vi "Force Control Parameters DAO.vi"(7 "Config Ref Number":T2, 8 "error in (no error)":errorcluster, 9 "Force Control Parameters In":T1, 11 "DAO Actions":T3) -> (0 "error out":errorcluster, 2 "Force Control Parameters Out":T1, 4 "Config Ref Number out":T2)   [LabVIEW 2013]
uses:
  Metadata/Persistant DAO Actions.ctl
  <vilib>/Utility/config.llb/Config Data RefNum.ctl
  Force Control Parameters.ctl
  <vilib>/Utility/config.llb/Write Key (Boolean).vi
  <vilib>/Utility/config.llb/Write Key (I32).vi
  <vilib>/Utility/config.llb/Read Key (Boolean).vi
  <vilib>/Utility/config.llb/Read Key (I32).vi
  <vilib>/Utility/config.llb/NI_LVConfig.lvlib
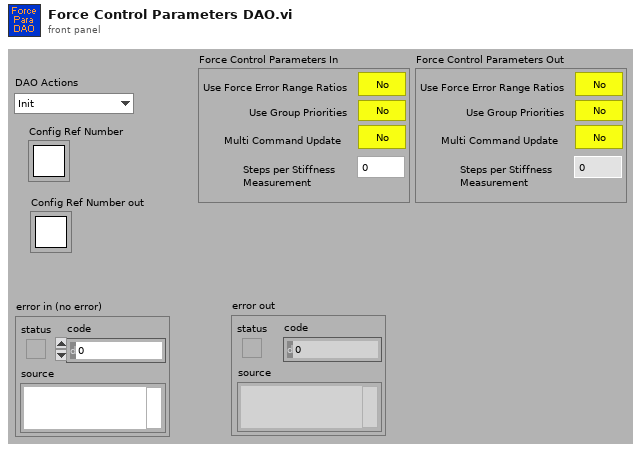
[diagram p1: front panel]
types:
  T1 = typedef "Force Control Parameters.ctl" = cluster{"Use Force Error Range Ratios":bool, "Use Group Priorities":bool, "Multi Command Update":bool, "Steps per Stiffness \nMeasurement":i32}
  T2 = typedef "NI_LVConfig.lvlib/Config Data RefNum.ctl" = refnum<k1>
  T3 = typedef "Persistant DAO Actions.ctl" = enum16{"Init", "Get", "Set", "Load", "Save"}
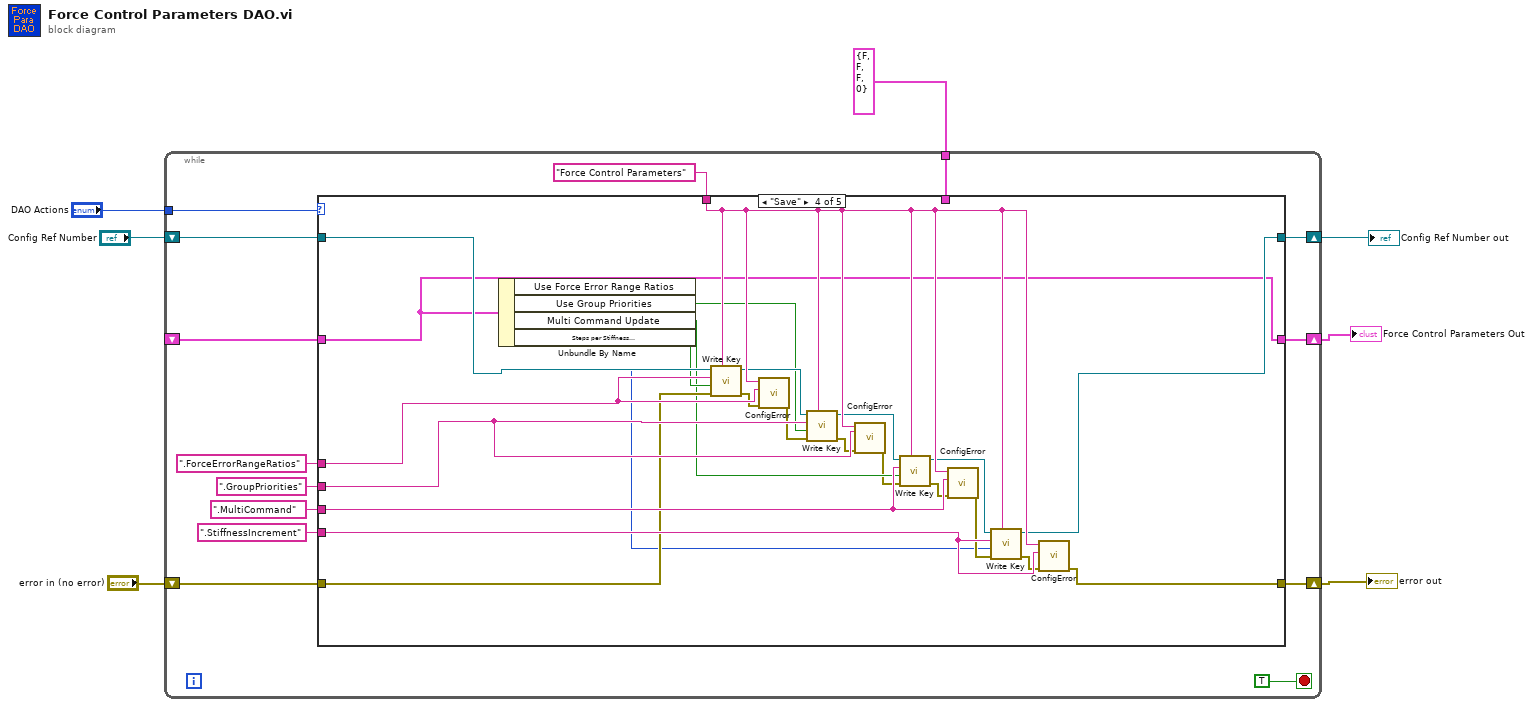
[diagram p0: block diagram]
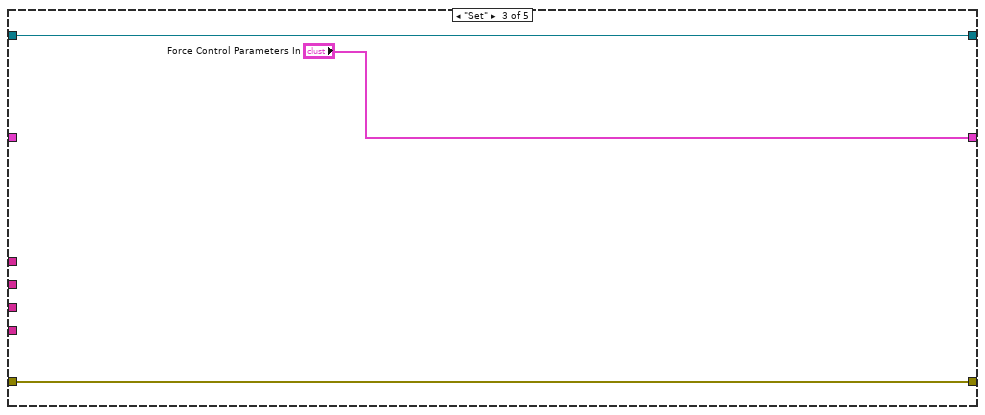
[diagram p4: hidden frame]
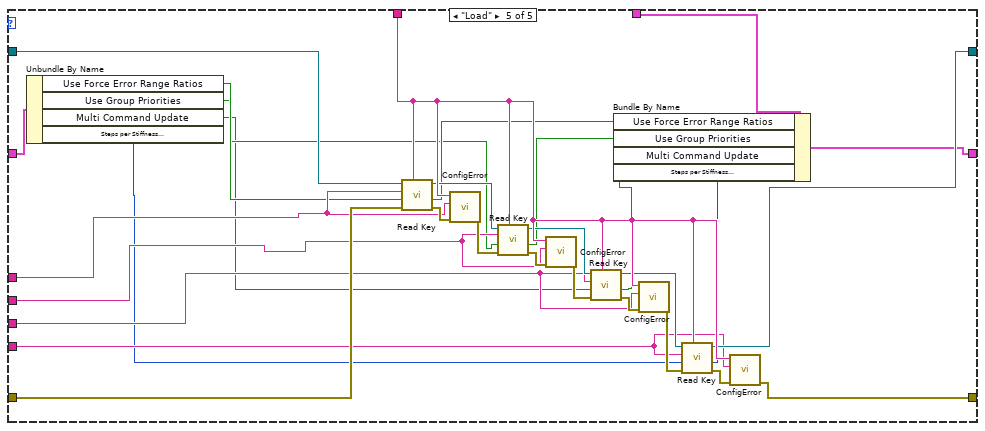
[diagram p5: hidden frame]
diagram:
  n1 = while {
    tunnel: "DAO Actions" -> [w20]
    shift-right: [w19] -> w1
    shift-left: _ -> [w18]
    shift-right: [w11] -> w2
    shift-left: "error in (no error)" -> [w13]
    shift-right: [w9] -> w4
    shift-left: "Config Ref Number" -> [w10]
    tunnel: T1 {"Use Force Error Range Ratios"=FALSE, "Use Group Priorities"=FALSE, "Multi Command Update"=FALSE, "Steps per Stiffness \nMeasurement"=0} ("Force Control Parameters In") -> [w8]
    stop <- TRUE stop-if-true
    n2 = case shown="\"Save\"" w20 {
      tunnel: [w24 w27 "Force Control Parameters In" w45 w60] -> w19
      tunnel: w18 -> [_ w27 _ w45 w59]
      tunnel: ".ForceErrorRangeRatios" ("string") -> [_ _ _ w54 w64]
      tunnel: ".GroupPriorities" ("string") -> [_ _ _ w53 w63]
      tunnel: ".MultiCommand" ("string") -> [_ _ _ w52 w62]
      tunnel: ".StiffnessIncrement" ("string") -> [_ _ _ w51 w61]
      tunnel: w13 -> [w22 w26 w28 w50 w84]
      tunnel: "Force Control Parameters" ("section") -> [_ _ _ w49 w83]
      tunnel: [w22 w26 w28 w48 w82] -> w11
      tunnel: w10 -> [w23 w25 w29 w47 w81]
      tunnel: [w23 w25 w29 w46 w80] -> w9
      tunnel: w8 -> [w24 _ _ _ w79]
      frame "Init" {
      }
      frame "Get" {
      }
      frame "Set" {
      }
      frame "Save" {
        n3 = Unbundle By Name(w45) -> ("Use Force Error Range Ratios"=w44:bool, "Use Group Priorities"=w40:bool, "Multi Command Update"=w36:bool, "Steps per Stiffness \nMeasurement"=w31:i32)
        n4 = call-poly <vilib>:"Write Key.vi"("section"=w49, "error in (no error)"=w50, "value"=w44, "key"=w54, "refnum"=w47) -> ("error out"=w43:errorcluster, "refnum out"=w41:T2)  [unwired: 4 in, 1 out]
        n5 = call "ConfigError.vi"("error in (no error)"=w43, "Key"=w54, "Section"=w49) -> ("error out"=w39:errorcluster)  [unwired: 8 in]
        n6 = call-poly <vilib>:"Write Key.vi"("section"=w49, "error in (no error)"=w39, "value"=w40, "key"=w53, "refnum"=w41) -> ("error out"=w42:errorcluster, "refnum out"=w37:T2)  [unwired: 4 in, 1 out]
        n7 = call "ConfigError.vi"("error in (no error)"=w42, "Key"=w53, "Section"=w49) -> ("error out"=w35:errorcluster)  [unwired: 8 in]
        n8 = call-poly <vilib>:"Write Key.vi"("section"=w49, "error in (no error)"=w35, "value"=w36, "key"=w52, "refnum"=w37) -> ("error out"=w38:errorcluster, "refnum out"=w33:T2)  [unwired: 4 in, 1 out]
        n9 = call "ConfigError.vi"("error in (no error)"=w38, "Key"=w52, "Section"=w49) -> ("error out"=w32:errorcluster)  [unwired: 8 in]
        n10 = call-poly <vilib>:"Write Key.vi"("section"=w49, "error in (no error)"=w32, "value"=w31, "key"=w51, "refnum"=w33) -> ("error out"=w34:errorcluster, "refnum out"=w46:T2)  [unwired: 4 in, 1 out]
        n11 = call "ConfigError.vi"("error in (no error)"=w34, "Key"=w51, "Section"=w49) -> ("error out"=w48:errorcluster)  [unwired: 8 in]
      }
      frame "Load" {
        n12 = Unbundle By Name(w59) -> ("Use Force Error Range Ratios"=w58:bool, "Use Group Priorities"=w57:bool, "Multi Command Update"=w56:bool, "Steps per Stiffness \nMeasurement"=w55:i32)
        n13 = call-poly <vilib>:"Read Key.vi"("section"=w83, "error in (no error)"=w84, "default value"=w58, "key"=w64, "refnum"=w81) -> ("error out"=w78:errorcluster, "value"=w68:bool, "refnum out"=w76:T2)  [unwired: 3 in, 1 out]
        n14 = call "ConfigError.vi"("error in (no error)"=w78, "Key"=w64, "Section"=w83) -> ("error out"=w75:errorcluster)  [unwired: 8 in]
        n15 = call-poly <vilib>:"Read Key.vi"("section"=w83, "error in (no error)"=w75, "default value"=w57, "key"=w63, "refnum"=w76) -> ("error out"=w77:errorcluster, "value"=w67:bool, "refnum out"=w73:T2)  [unwired: 3 in, 1 out]
        n16 = call "ConfigError.vi"("error in (no error)"=w77, "Key"=w63, "Section"=w83) -> ("error out"=w72:errorcluster)  [unwired: 8 in]
        n17 = call-poly <vilib>:"Read Key.vi"("section"=w83, "error in (no error)"=w72, "default value"=w56, "key"=w62, "refnum"=w73) -> ("error out"=w74:errorcluster, "value"=w66:bool, "refnum out"=w70:T2)  [unwired: 3 in, 1 out]
        n18 = call "ConfigError.vi"("error in (no error)"=w74, "Key"=w62, "Section"=w83) -> ("error out"=w69:errorcluster)  [unwired: 8 in]
        n19 = call-poly <vilib>:"Read Key.vi"("section"=w83, "error in (no error)"=w69, "default value"=w55, "key"=w61, "refnum"=w70) -> ("error out"=w71:errorcluster, "value"=w65:i32, "refnum out"=w80:T2)  [unwired: 3 in, 1 out]
        n20 = Bundle By Name(cluster=w79, "Use Force Error Range Ratios"=w68, "Use Group Priorities"=w67, "Multi Command Update"=w66, "Steps per Stiffness \nMeasurement"=w65) -> (w60:T1)
        n21 = call "ConfigError.vi"("error in (no error)"=w71, "Key"=w61, "Section"=w83) -> ("error out"=w82:errorcluster)  [unwired: 8 in]
      }
    }
  }
  "error out" <- w2
  "Config Ref Number out" <- w4
  "Force Control Parameters Out" <- w1
